vi "circular_calc_bounds.vi"(9 "Lower Bound":dbl, 10 "Upper Bound":dbl, 11 "Desired Position":dbl) -> (3 "Desired Position Out":dbl)   [LabVIEW 2012]
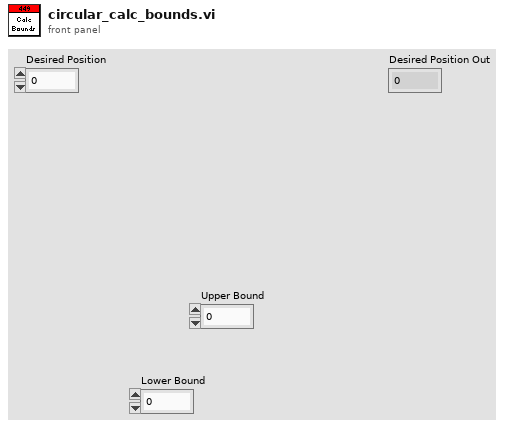
[diagram p1: front panel]
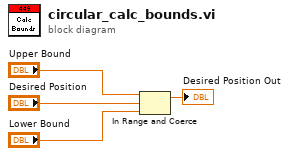
[diagram p0: block diagram]
diagram:
  n1 = In Range and Coerce(upper limit="Upper Bound", x="Desired Position", lower limit="Lower Bound") -> (coerced(x)=→"Desired Position Out":dbl)  [unwired: 1 out]
